vi "Call Subpanel VI.vi"(8 "error in (no error)":errorcluster, 10 "VI Refnum":refnum<vi>, 11 "monitor configuration in":refnum<class "CCD monitor configuration.lvclass">) -> (0 "error out":errorcluster, 3 "monitor configuration out":refnum<class "CCD monitor configuration.lvclass">)   [LabVIEW 2016, in "CCD monitor.lvlib" / "CCD monitor configuration.lvclass"]
uses:
  <userlib>/Common Components/Hardware/Abstract System/Monitor/CCD monitor configuration.lvclass
  <userlib>/Configuration Dialog Actor/Configuration.lvclass
  C:/Program Files (x86)/National Instruments/LabVIEW 2016/user.lib/Configuration Dialog Actor/Configuration.lvclass
  <userlib>/Configuration Dialog Actor/Configuration.lvclass/Configuration.ctl
  <vilib>/Utility/error.llb/Error Cluster From Error Code.vi
  <vilib>/ErrorRing/Error Ring.xnode
  <userlib>/Common Components/Hardware/CCD/CCD Configuration.lvclass
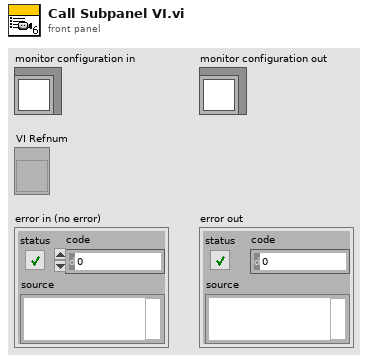
[diagram p1: front panel]
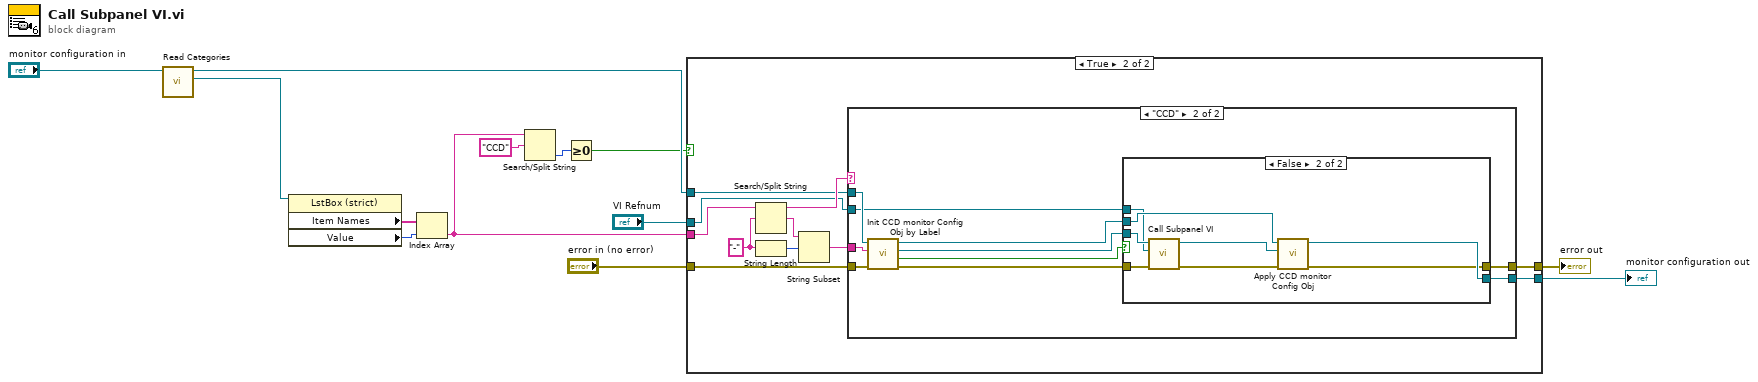
[diagram p0: block diagram]
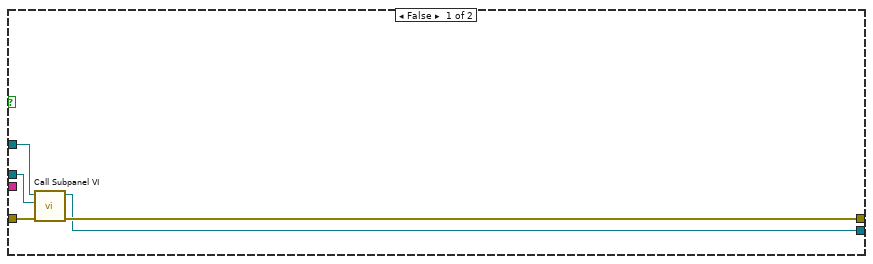
[diagram p2: hidden frame]
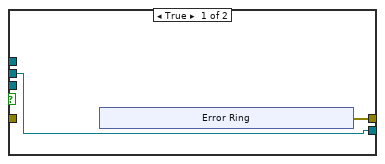
[diagram p4: hidden frame]
diagram:
  n1 = call <userlib>:"Read Categories.vi"("Configuration in"="monitor configuration in") -> ("Categories"=w12:refnum<vi>, "Configuration out"=w9:refnum<class "CCD monitor configuration.lvclass">)  [unwired: 8 in, 1 out]
  n2 = property class="LstBox (strict)"(reference=w12) -> ("Item Names"=w10:string[], "Value"=w11:i32)  [unwired: 1 in, 2 out]
  n3 = Index Array(array=w10, index=w11) -> (element=w4:string)
  n4 = Search/Split String(string=w4, search string/char (-)="CCD") -> (offset of match=w1:i32)  [unwired: 1 in, 2 out]
  n5 = Greater Or Equal To 0?(x=w1) -> (x >= 0?=w3:bool)
  n6 = case shown="True" w3 {
    tunnel: [w18 w21] -> w5
    tunnel: [w17 w22] -> w6
    tunnel: w9 -> [w16 w24]
    tunnel: "VI Refnum" -> [w15 w19]
    tunnel: "error in (no error)" -> [w14 w23]
    tunnel: w4 -> [_ w29]
    frame False {
      n7 = call-parent "Call Subpanel VI.vi"("error in (no error)"=w14, "VI Refnum"=w15, "Configuration in"=w16) -> ("error out"=w18:errorcluster, "Configuration out"=w17:refnum<class "CCD monitor configuration.lvclass">)  [unwired: 7 in]
    }
    frame True {
      w28 = "-" ("search string/char (-)")
      n8 = Search/Split String(string=w29, search string/char (-)=w28) -> (substring before match=w25:string, match + rest of string=w26:string)  [unwired: 1 in, 1 out]
      n9 = String Length(string=w28) -> (length=w27:i32)
      n10 = String Subset(string=w26, offset (0)=w27) -> (substring=w20:string)  [unwired: 1 in]
      n11 = case shown="\"CCD\"" w25 {
        tunnel: w24 -> [w31 w41]
        tunnel: w23 -> [w30 w39]
        tunnel: [w31 w34] -> w22
        tunnel: [w30 w33] -> w21
        tunnel: w20 -> [_ w40]
        tunnel: w19 -> [_ w36]
        frame Default {
        }
        frame "CCD" {
          n12 = call <userlib>:"Init CCD monitor Config Obj by Label.vi"("error in (no error)"=w39, "Label"=w40, "Hardware.lvlib:CCD monitor.lvlib:CCD monitor configuration.lvclass"=w41) -> ("error out"=w35:errorcluster, "not found?"=w32:bool, "Hardware.lvlib:CCD.lvlib:CCD Configuration.lvclass"=w37:refnum<class "CCD Configuration.lvclass">, "reference out"=w38:refnum<class "CCD monitor configuration.lvclass">)  [unwired: 5 in]
          n13 = case shown="False" w32 {
            tunnel: w38 -> [w43 w55]
            tunnel: w37 -> [_ w54]
            tunnel: w36 -> [_ w53]
            tunnel: w35 -> [_ w52]
            tunnel: [w43 w51] -> w34
            tunnel: [w42 w50] -> w33
            frame True {
              n14 = xnode "Error Ring"() -> ("error out"=w42:errorcluster)
            }
            frame False {
              n15 = call-dynamic "Call Subpanel VI.vi"("error in (no error)"=w52, "VI Refnum"=w53, "CCD Configuration in"=w54) -> ("error out"=w48:errorcluster, "CCD Configuration out"=w49:refnum<class "CCD Configuration.lvclass">)  [unwired: 7 in]
              n16 = call <userlib>:"Apply CCD monitor Config Obj.vi"("error in (no error)"=w48, "Hardware.lvlib:CCD.lvlib:CCD Configuration.lvclass"=w49, "Hardware.lvlib:CCD monitor.lvlib:CCD monitor configuration.lvclass"=w55) -> ("error out"=w50:errorcluster, "Hardware.lvlib:CCD monitor.lvlib:CCD monitor configuration.lvclass 2"=w51:refnum<class "CCD monitor configuration.lvclass">)  [unwired: 7 in]
            }
          }
        }
      }
    }
  }
  "error out" <- w5
  "monitor configuration out" <- w6
